vi "Reverse & Rotate String Part 7.vi"() -> ()   [LabVIEW 2020]
panel:
  out "first char last":string
  out "reversed":string
  in  "string":string
  # "Reverse & Rotate String"
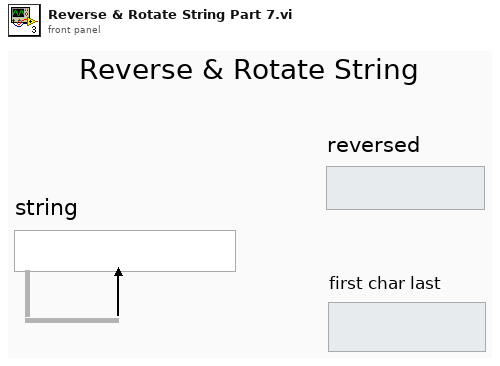
[diagram p1: front panel]
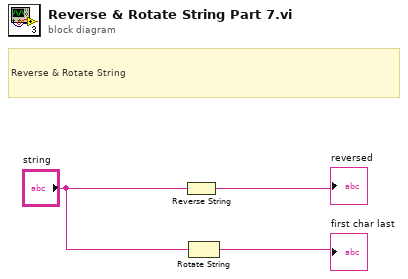
[diagram p0: block diagram]
diagram:
  # "Reverse & Rotate String"
  n1 = Reverse String(1:"string") -> (0:→"reversed":string)
  n2 = Rotate String(1:"string") -> (0:→"first char last":string)
